vi "latch variable panel event structure test.vi"() -> ()   [LabVIEW 2010]
panel:
  out "num events":i16
  out "num presses":i16
  in  "stop":bool
  in  "OK Button":bool
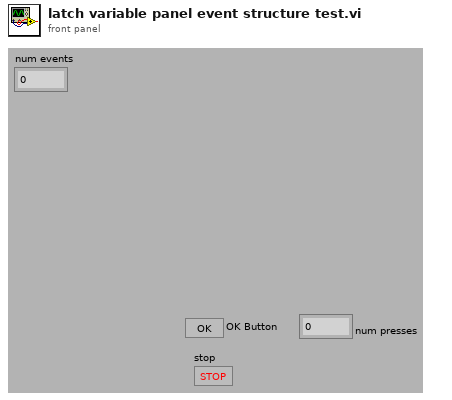
[diagram p1: front panel]
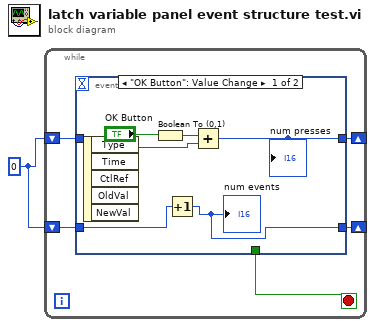
[diagram p0: block diagram]
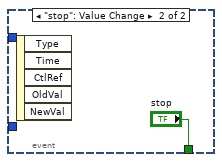
[diagram p2: hidden frame]
diagram:
  w1 = i16 0 ("Numeric")
  n1 = while {
    shift-right: [w6] -> _
    shift-left: w1 -> [w5]
    shift-right: [w3] -> _
    shift-left: w1 -> [w4]
    stop <- w2 stop-if-true
    n2 = event shown="[0] \"OK Button\": Value Change" {
      selector: _ -> [_ _]
      dyn-events: _ -> [_ _]
      timeout: _ -> [_ _]
      tunnel: [w10 _] -> w6
      tunnel: w5 -> [w9 _]
      tunnel: w4 -> [w8 _]
      tunnel: [w7 _] -> w3
      tunnel: [_ "stop"] -> w2
      event "OK Button": Value Change {
        n3 = event-data() -> ()  [unwired: 1 in, 5 out]
        n4 = Boolean To (0,1)(Boolean="OK Button") -> (0, 1=w11:i16)
        n5 = Increment(x=w8) -> (x+1=w7:i16)
        "num events" <- w7
        n6 = Add(x=w11, y=w9) -> (x+y=w10:i16)
        "num presses" <- w10
      }
      event "stop": Value Change {
        n7 = event-data() -> ()  [unwired: 1 in, 5 out]
      }
    }
  }
